vi "Resistance Measuring 2400.vi"() -> ()   [LabVIEW 2022 SP3]
uses:
  2022 MPhys Project/Keithley 24XX Sweep and Acquire Measurements Folder/Public/Data/Read (Single Point).vi
  2022 MPhys Project/Keithley 24XX Sweep and Acquire Measurements Folder/Keithley 24XX.lvlib
panel:
  out "Resistance":dbl
  out "Volt":sgl[](array[numeric])
  out "Current":sgl[](array[numeric])
  in  "Current micro amps":dbl
  in  "Serial Configuration":T1={"Baud Rate"=9600, "Parity"=0, "Data Bits"=8, "Stop Bits"=10, "Flow Control"=0, "VISA resource name"=""} {"Flow Control" items=["None", "XON/XOFF", "RTS/CTS", "XON/XOFF & RTS/CTS", "DTR/DSR", "XON/XOFF & DTR/DSR"]; "Stop Bits" items=["1.0"=10, "1.5"=15, "2.0"=20]; "Data Bits" items=["7"=7, "8"=8]; "Parity" items=["None", "Odd", "Even", "Mark", "Space"]; "Baud Rate" items=["300"=300, "600"=600, "1200"=1200, "2400"=2400, "4800"=4800, "9600"=9600, "19200"=19200]}
  in  "Enable Current Auto Range (T:Enable)":bool=TRUE
  in  "Current Manual Range (1.0)":dbl=1.0
  in  "Compliance  Level (0.1)":dbl=0.1
  in  "Source Mode  (0: Voltage)":u16(ring) items=["Voltage", "Current"]
  in  "Number of measurement repeats":dbl
  # "Measurement Values"
  # "Source meter"
  # "Configure Measurements"
  # "Choosing Current To Input"
  # "Configure Measurements"
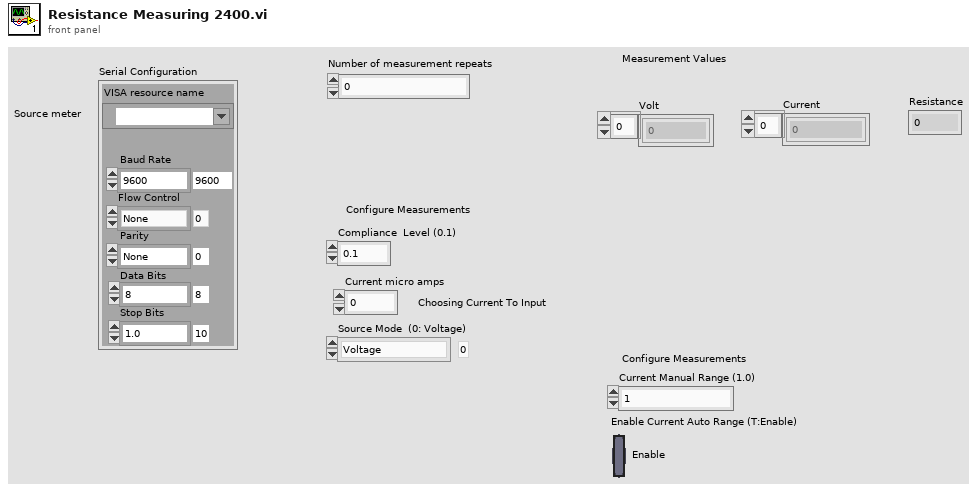
[diagram p1: front panel]
types:
  T1 = cluster{"Baud Rate":u32, "Parity":u16, "Data Bits":u16, "Stop Bits":u16, "Flow Control":u16, "VISA resource name":refnum<visa-resource-name>}
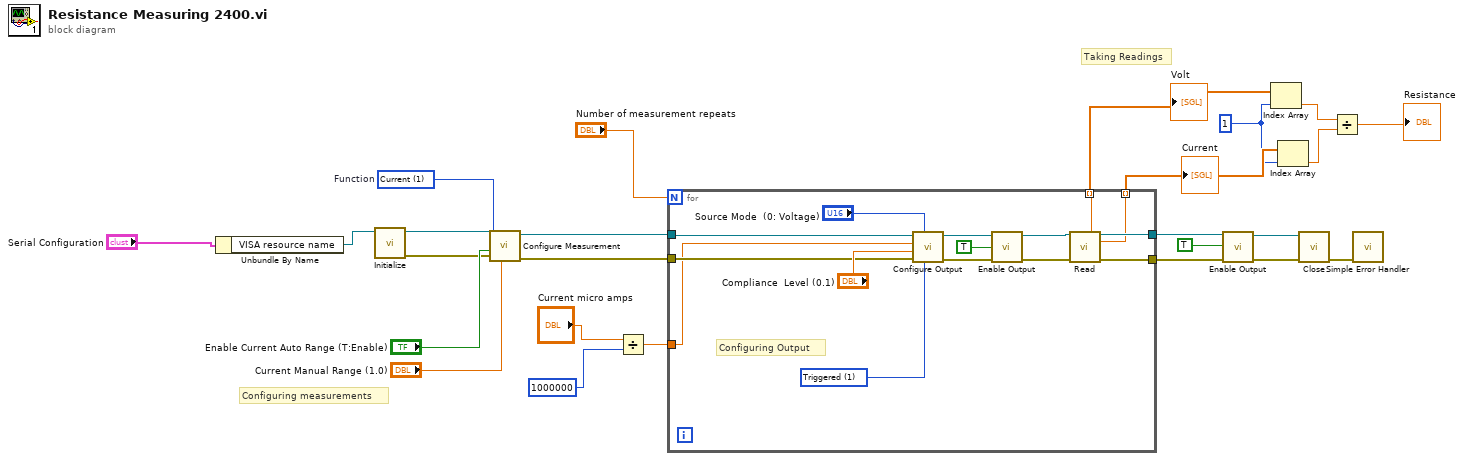
[diagram p0: block diagram]
diagram:
  w4 = 1
  w25 = u16 1 items=["Volts", "Current", "Resistance"]  # Function
  # "Taking Readings"
  # "Configuring measurements"
  n1 = Unbundle By Name("Serial Configuration") -> ("VISA resource name"=w18:refnum<visa-resource-name>)
  n2 = call "Initialize.vi"("VISA resource name"=w18) -> ("error out"=w11:errorcluster, "VISA resource name out"=w12:refnum<visa-resource-name>)  [unwired: 9 in]
  n3 = call "Configure Measurement.vi"("Manual Range (1.0)"="Current Manual Range (1.0)", "error in (no error)"=w11, "Enable Auto Range (T:Enable)"="Enable Current Auto Range (T:Enable)", "Function (0: Volts)"=w25, "VISA resource name"=w12) -> ("error out"=w13:errorcluster, "VISA resource name out"=w14:refnum<visa-resource-name>)  [unwired: 5 in]
  n4 = Divide(x="Current micro amps", y=1000000) -> (x/y=w8:dbl)
  n5 = for {
    N: "Number of measurement repeats" -> [_]
    tunnel: [w34] -> w16
    tunnel: [w33] -> w17
    tunnel: w14 -> [w32]
    tunnel: w13 -> [w31]
    tunnel: w8 -> [w28]
    tunnel: [w27] -> w5 mode=indexing
    tunnel: [w26] -> w6 mode=indexing
    w29 = u16 1 items=["Immediate", "Triggered"] ("Output Type  (0: Immediate)")
    # "Configuring Output"
    n6 = call "Configure Output.vi"("Output Type  (0: Immediate)"=w29, "Source Mode  (0: Voltage)"="Source Mode  (0: Voltage)", "error in (no error)"=w31, "Compliance  Level (0.1)"="Compliance  Level (0.1)", "Output Level (0)"=w28, "VISA resource name"=w32) -> ("error out"=w35:errorcluster, "VISA resource name out"=w36:refnum<visa-resource-name>)  [unwired: 4 in]
    n7 = call "Enable Output.vi"("error in (no error)"=w35, "Enable Output (T: Enable)"=TRUE, "VISA resource name"=w36) -> ("error out"=w37:errorcluster, "VISA resource name out"=w38:refnum<visa-resource-name>)  [unwired: 7 in]
    n8 = call-poly "Read.vi"("VISA resource name"=w38, "error in (no error)"=w37) -> ("Voltage"=w26:sgl, "VISA resource name out"=w33:refnum<visa-resource-name>, "Current"=w27:sgl, "error out"=w34:errorcluster)  [unwired: 7 in, 3 out]
  }
  "Current" <- w5
  "Volt" <- w6
  n9 = call "Enable Output.vi"("error in (no error)"=w16, "Enable Output (T: Enable)"=TRUE, "VISA resource name"=w17) -> ("error out"=w21:errorcluster, "VISA resource name out"=w22:refnum<visa-resource-name>)  [unwired: 7 in]
  n10 = Index Array(array=w6, index=w4) -> (element=w3:sgl)
  n11 = Index Array(array=w5, index=w4) -> (element=w2:sgl)
  n12 = call "Close.vi"("error in (no error)"=w21, "VISA resource name"=w22) -> ("error out"=w15:errorcluster)  [unwired: 9 in]
  n13 = Divide(x=w3, y=w2) -> (x/y=→"Resistance":sgl)
  n14 = call <vilib>:"Simple Error Handler.vi"("error in (no error)"=w15) -> ()  [unwired: 4 in, 5 out]
